vi "crio_RT.vi"() -> ()   [LabVIEW 2019]
uses:
  <vilib>/Platform/TimedLoop/XDataNode/timing_clust.ctl
  <vilib>/Platform/TimedLoop/XDataNode/nitl_modes.ctl
  <vilib>/Platform/TimedLoop/XDataNode/wakeup.ctl
  <vilib>/FPGAPlugInAG/cRIO-9054/niLvFpga_Open_cRIO-9054.vi
  <vilib>/rvi/interface/common/dynamic/niFpgaDynamicAddResources.vi
  <vilib>/FPGAPlugInAG/Dynamic/niLvFpga_Run_Dynamic.vi
  <vilib>/Utility/error.llb/Error Cluster From Error Code.vi
  <vilib>/rvi/errors/niLvFpgaAdjustHostInterfaceError.vi
  <vilib>/FPGAPlugInAG/Dynamic/niLvFpga_Close_Dynamic.vi
  <vilib>/platform/TimedLoop/XDataNode/XDataNode.xnode
  <vilib>/rvi/interface/nirviOpenFPGA/nirviOpenFPGA.xnode
  FPGA Bitfiles/newwindtunnel_FPGATarget_test_X65+PG5pTZc.lvbitx
  <vilib>/rvi/interface/nirviMethod/nirviMethod.xnode
  <vilib>/rvi/interface/nirviReadWriteControl/nirviReadWriteControl.xnode
  <vilib>/rvi/interface/nirviCloseFPGA/nirviCloseFPGA.xnode
  <vilib>/Platform/TimedLoop/XDataNode/XDNodeRunTimeDep.lvlib
  <vilib>/ptbypt/NI_PtbyPt.lvlib
  NiFpgaLv.dll
  <vilib>/rvi/interface/Simulation/niFpgaSimulationCallBeginRW.vi
panel:
  in  "stop":bool
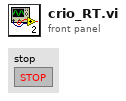
[diagram p1: front panel]
types:
  T1 = typedef "XDNodeRunTimeDep.lvlib/timing_clust.ctl" = cluster{"Expected End [f-1]":u64, "Actual End [f-1]":u64, "Finished Late? [f-1]":bool, "Expected End [i-1]":u64, "Actual End [i-1]":u64, "Finished Late? [i-1]":bool, "Expected Start [i]":u64, "Actual Start [i]":u64, "Expected Start [f]":u64, "Actual Start [f]":u64, "Source Name":string, "Structure Name":string, "Period":i64, "Deadline":i64, "Offset":i64, "Start":i64, "Priority":i32, "Timeout":i32, "Mode":T2, "Wakeup Reason":T3, "Error":errorcluster, "Source Type":string, "Secondary Source Type":string, "Global End Time":u64, "Global Start Time":u64, "Frame Duration":u64, "Iteration Duration":u64, "Assigned CPU":i32, "I/O Scan Engine Mode":u32}
  T2 = typedef "XDNodeRunTimeDep.lvlib/nitl_modes.ctl" = enum32{"No Change", "Process missed periods, maintain original phase", "Discard missed periods, maintain original phase", "Process missed periods, ignore original phase", "Discard missed periods, ignore original phase"}
  T3 = typedef "XDNodeRunTimeDep.lvlib/wakeup.ctl" = enum32{"Normal", "Aborted", "Asynchronous wakeup", "Timing source error", "Timed loop error", "Timeout"}
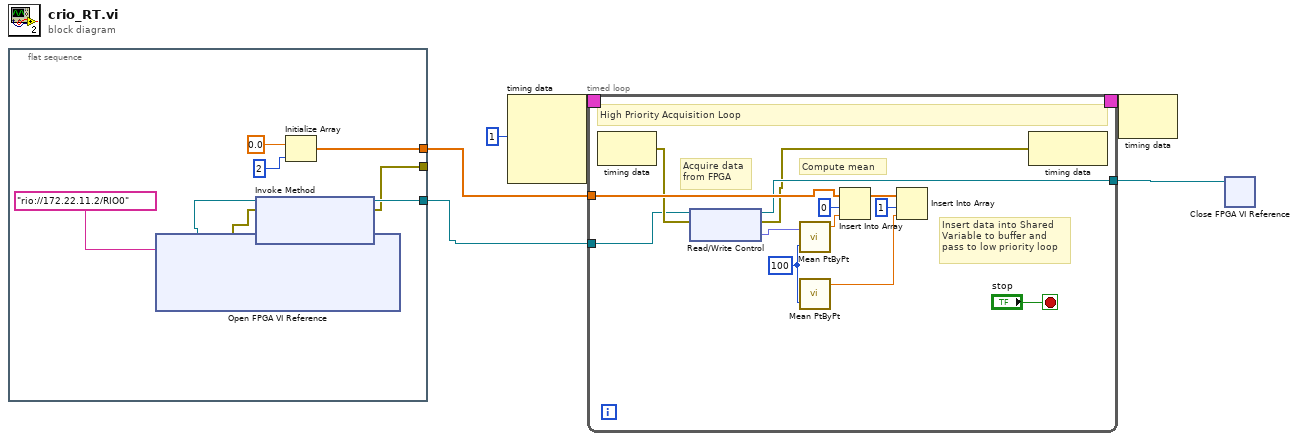
[diagram p0: block diagram]
diagram:
  n1 = flat-sequence {
    tunnel: [w14] -> w4
    tunnel: [w13] -> _
    tunnel: [w10] -> w2
    frame #0 {
      n2 = xnode "Open FPGA VI Reference"("resource name"=tag "rio://172.22.11.2/RIO0") -> ("FPGA VI Reference Out"=w9:refnum<k20>, "error out"=w8:errorcluster)  [unwired: 1 in]
      n3 = xnode "Invoke Method"("FPGA VI Reference In"=w9, "error in"=w8) -> ("FPGA VI Reference Out"=w14:refnum<k20>, "error out"=w13:errorcluster)  [unwired: 1 in]
      n4 = Initialize Array(0.0 ("AI3"), 2 ("dimension size")) -> (w10:dbl[])
    }
  }
  n5 = node-c288(i64 1 ("Period")) -> (w6:T1)  [unwired: 3 in]
  n6 = timed-loop {
    timing: w6 -> [_]
    timing-out: [_] -> w5
    tunnel: w4 -> [w19]
    tunnel: [w18] -> w3
    tunnel: w2 -> [w21]
    stop <- "stop" stop-if-true
    w26 = 100 ("sample length")
    # "Compute mean"
    # "Insert data into Shared \nVariable to buffer and \npass to low priority loop"
    # "Acquire data\nfrom FPGA"
    # "High Priority Acquisition Loop"
    n7 = node-c288() -> (w20:errorcluster)  [unwired: 1 in]
    n8 = xnode "Read/Write Control"("FPGA VI Reference In"=w19, "error in"=w20) -> ("FPGA VI Reference Out"=w18:refnum<k20>, "error out"=w17:errorcluster, "Mod3/AI0"=w15:fxp<+/-,24,5>)
    n9 = call <vilib>:"Mean PtByPt.vi"("x"=w15, "sample length"=w26) -> ("mean"=w27:dbl)  [unwired: 2 in, 1 out]
    n10 = call <vilib>:"Mean PtByPt.vi"("sample length"=w26) -> ("mean"=w24:dbl)  [unwired: 3 in, 1 out]
    n11 = Insert Into Array(array=w21, index=0, new element=w27) -> (w25:dbl[])
    n12 = Insert Into Array(array=w25, index=1, new element=w24) -> ()  [unwired: 1 out]
    n13 = node-c288(w17) -> ()  [unwired: 1 out]
  }
  n14 = node-c288(w5) -> ()  [unwired: 1 out]
  n15 = xnode "Close FPGA VI Reference"("FPGA VI Reference In"=w3) -> ()  [unwired: 1 in, 1 out]
